vi "Send TV.vi"(8 "error in (no error)":errorcluster, 11 "Model in":refnum<class "Model.lvclass">) -> (0 "error out":errorcluster, 3 "Model out":refnum<class "Model.lvclass">)   [LabVIEW 2015, in "Model.lvclass"]
uses:
  Model.lvclass
  Typedefs/Cylinder Results.ctl
  Model.lvclass/Model.ctl
  Calculators/Percentage To Turbo Valve Voltage/Percentage To Turbo Valve Voltage.lvclass
  DAQmx/DAQmx.lvclass
  Typedefs/FAMT Typedefs.lvlib
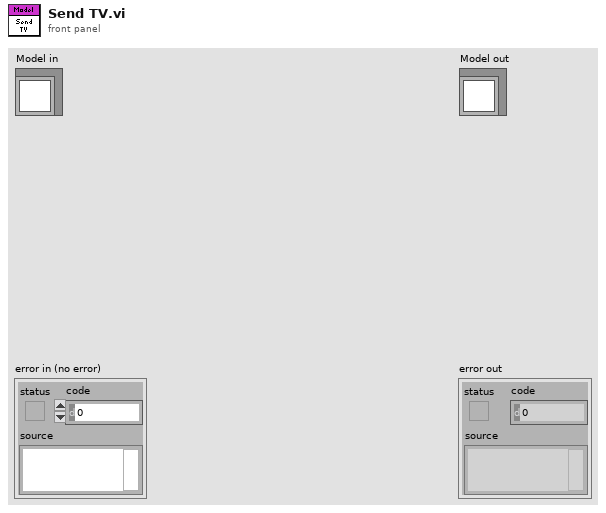
[diagram p1: front panel]
types:
  T1 = typedef "FAMT Typedefs.lvlib/Cylinder Results.ctl" = cluster{"PSV1 Value":dbl[unit], "PSV2 Value":dbl[unit], "TV Value":dbl[unit]}
  T2 = typedef "FAMT Typedefs.lvlib/Turbo Valve Settings.ctl" = cluster{"Bias":dbl, "Minimum Voltage":dbl, "Maximum Voltage":dbl, "Off Value":dbl}
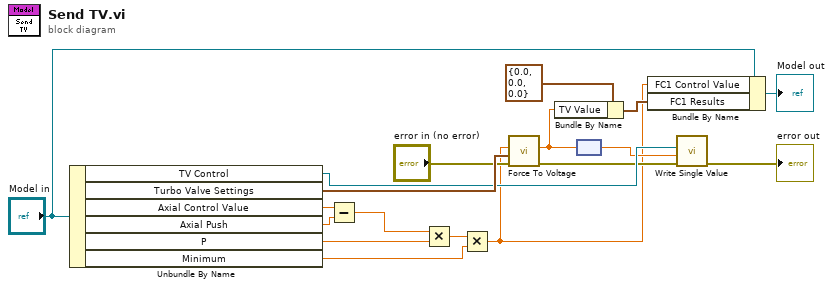
[diagram p0: block diagram]
diagram:
  n1 = Unbundle By Name("Model in") -> ("TV Control"=w15:refnum<k21>, "Turbo Valve Settings"=w16:T2, "Axial Control Value"=w13:dbl, "Axial Push"=w12:dbl, "P"=w3:dbl, "Minimum"=w2:dbl)
  n2 = Subtract(x=w13, y=w12) -> (x-y=w1:dbl)
  n3 = Multiply(x=w1, y=w3) -> (x*y=w5:dbl)
  n4 = Multiply(x=w5, y=w2) -> (x*y=w4:dbl)
  n5 = call "Force To Voltage.vi"("error in (no error)"="error in (no error)", "Turbo Valve Settings"=w16, "Percentage"=w4) -> ("error out"=w14:errorcluster, "Voltage"=w7:dbl[unit])  [unwired: 6 in, 1 out]
  n6 = Bundle By Name(cluster=T1 {"PSV1 Value"=0.0, "PSV2 Value"=0.0, "TV Value"=0.0} ("FC1 Results"), "TV Value"=w7) -> (w9:T1)
  n7 = node(w7) -> (w8:dbl)
  n8 = Bundle By Name(cluster="Model in", "FC1 Control Value"=w4, "FC1 Results"=w9) -> (→"Model out":refnum<class "Model.lvclass">)
  n9 = call "Write Single Value.vi"("error in (no error)"=w14, "Value"=w8, "Channel"=w15) -> ("error out"=→"error out":errorcluster)  [unwired: 7 in, 1 out]
